vi "Transform LIDAR Data.vi"(8 "New Orientation (X m, Y m, T rad)":dbl[](array[numeric]), 9 "Orientation (X m, Y m, T rad)":dbl[](array[numeric]), 10 "Direction (deg)":dbl[](array[numeric]), 11 "Magnitude (mm)":dbl[](array[numeric])) -> (0 "New Orientation (X m, Y m, T rad) out":dbl[](array[numeric]), 2 "Direction out (rad)":dbl[](array[numeric]), 3 "Magnitude out (m)":dbl[](array[numeric]))   [LabVIEW 2017]
uses:
  <vilib>/Analysis/coordinate.llb/2D Cartesian Coordinate Rotation (Scalar).vi
  <vilib>/Analysis/coordinate.llb/2D Cartesian Coordinate Shift (Array).vi
  <vilib>/Utility/AngleManip/Degrees to Radians (Scalar DBL).vi
  <vilib>/Analysis/NI_AALPro.lvlib
  <vilib>/Utility/AngleManip/NI_AngleManipulation.lvlib
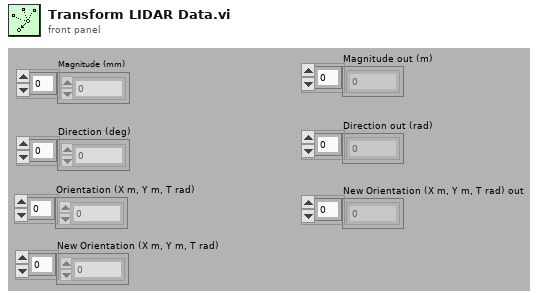
[diagram p1: front panel]
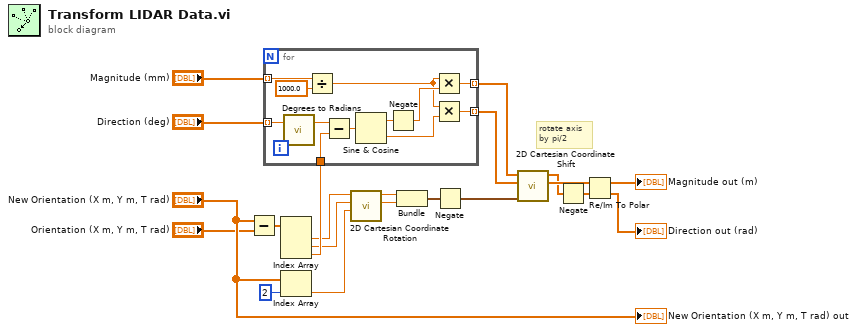
[diagram p0: block diagram]
diagram:
  # "rotate axis\nby pi/2"
  n1 = Subtract(x="New Orientation (X m, Y m, T rad)", y="Orientation (X m, Y m, T rad)") -> (x-y=w11:dbl[])
  n2 = Index Array(array=w11) -> (element #1=w8:dbl, element #2=w9:dbl, element #3=w10:dbl)  [unwired: 3 in]
  n3 = for {
    tunnel: "Direction (deg)" -> [w23] mode=indexing
    tunnel: "Magnitude (mm)" -> [w28] mode=indexing
    tunnel: w10 -> [w33]
    tunnel: [w27] -> w12 mode=indexing
    tunnel: [w26] -> w13 mode=indexing
    n4 = call-poly <vilib>:"Degrees to Radians.vi"("angle (deg)"=w23) -> ("angle (rad)"=w22:dbl)  [unwired: 2 in]
    n5 = Divide(x=w28, y=1000.0) -> (x/y=w25:dbl)
    n6 = Subtract(x=w22, y=w33) -> (x-y=w32:dbl)
    n7 = Sine & Cosine(0:w32) -> (1:w31:dbl, 2:w29:dbl)
    n8 = Negate(x=w31) -> (-x=w30:dbl)
    n9 = Multiply(x=w25, y=w30) -> (x*y=w27:dbl)
    n10 = Multiply(x=w25, y=w29) -> (x*y=w26:dbl)
  }
  n11 = Index Array(array="New Orientation (X m, Y m, T rad)", index=2) -> (element=w20:dbl)
  n12 = call-poly <vilib>:"2D Cartesian Coordinate Rotation.vi"("theta"=w20, "y"=w9, "x"=w8) -> ("y out"=w15:dbl, "x out"=w14:dbl)  [unwired: 6 in, 1 out]
  n13 = Bundle("x out"=w14, "y out"=w15) -> (w16:cluster{"x out":dbl, "y out":dbl})  [unwired: 1 in]
  n14 = Negate(x=w16) -> (-x=w2:cluster{"x out":dbl, "y out":dbl})
  n15 = call-poly <vilib>:"2D Cartesian Coordinate Shift.vi"("shift"=w2, "Y"=w13, "X"=w12) -> ("Y Out"=w18:dbl[], "X Out"=w17:dbl[])  [unwired: 6 in, 1 out]
  n16 = Negate(x=w17) -> (-x=w19:dbl[])
  n17 = Re/Im To Polar(2:w19, 3:w18) -> (0:→"Direction out (rad)":dbl[], 1:→"Magnitude out (m)":dbl[])
  "New Orientation (X m, Y m, T rad) out" <- "New Orientation (X m, Y m, T rad)"
